vi "Get Signal Classification.vi"(8 "error in (no error)":errorcluster, 11 "IO Class in":refnum<class "Signal.lvclass">) -> (0 "error out":errorcluster, 2 "Classification":string, 3 "IO Class out":refnum<class "Signal.lvclass">)   [LabVIEW 2015, in "Signal.lvclass"]
uses:
  Signal.lvclass
  Configuration.ctl
  Read Configuration.vi
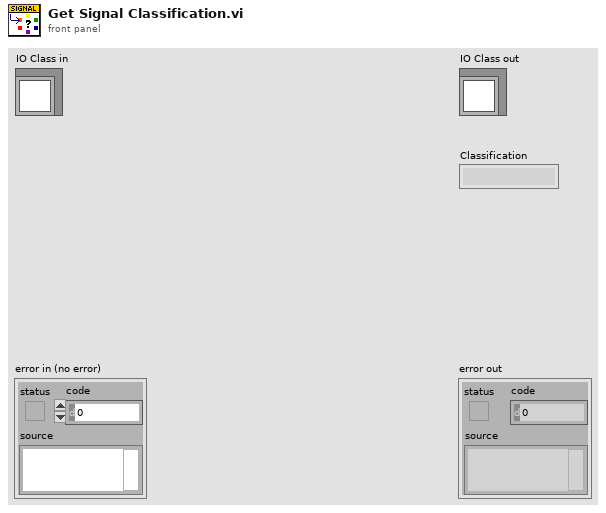
[diagram p1: front panel]
types:
  T1 = typedef "Signal.lvclass/Configuration.ctl" = cluster{"Classification":string, "Direction":string, "Type":string}
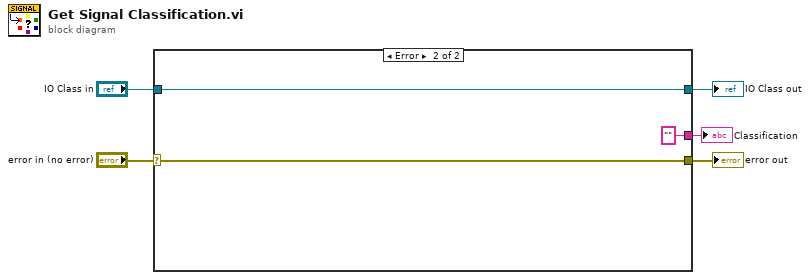
[diagram p0: block diagram]
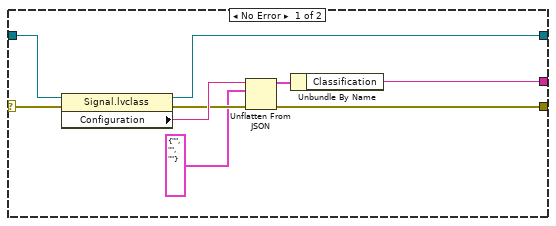
[diagram p2: hidden frame]
diagram:
  n1 = case shown="Error" "error in (no error)" {
    selector: "error in (no error)" -> [w10 w17]
    tunnel: [w7 w17] -> w4
    tunnel: [w8 w16] -> w2
    tunnel: "IO Class in" -> [w9 w16]
    tunnel: [w6 "" ("Classification")] -> w1
    frame No Error {
      n2 = property class="Signal.lvclass"(reference=w9, error in=w10) -> (reference out=w8:refnum<class "Signal.lvclass">, error out=w13:errorcluster, "Configuration"=w14:string)
      n3 = Unflatten From JSON(JSON string=w14, type and defaults=T1 {"Classification"="", "Direction"="", "Type"=""} ("Configuration"), error in (no error)=w13) -> (value=w12:T1, error out=w7:errorcluster)  [unwired: 4 in]
      n4 = Unbundle By Name(w12) -> ("Classification"=w6:string)
    }
    frame Error {
    }
  }
  "error out" <- w4
  "IO Class out" <- w2
  "Classification" <- w1
